vi "GetVIByName.vi"(0 "Application Ref in":refnum<vi>, 5 "VI Name":string, 7 "Timeout(5 sec)":dbl=5.0, 11 "error in (no error)":errorcluster) -> (4 "Application Ref out":refnum<vi>, 6 "VI Reference":refnum<vi>, 15 "error out":errorcluster)   [LabVIEW 2016, in "Drona.lvlib" / "GetVI.lvlib"]
doc: "Gives the reference of the specified VI given by VI name as input."
uses:
  GetVI.lvlib
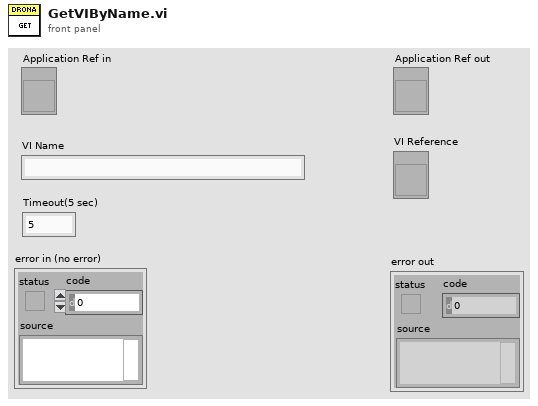
[diagram p1: front panel]
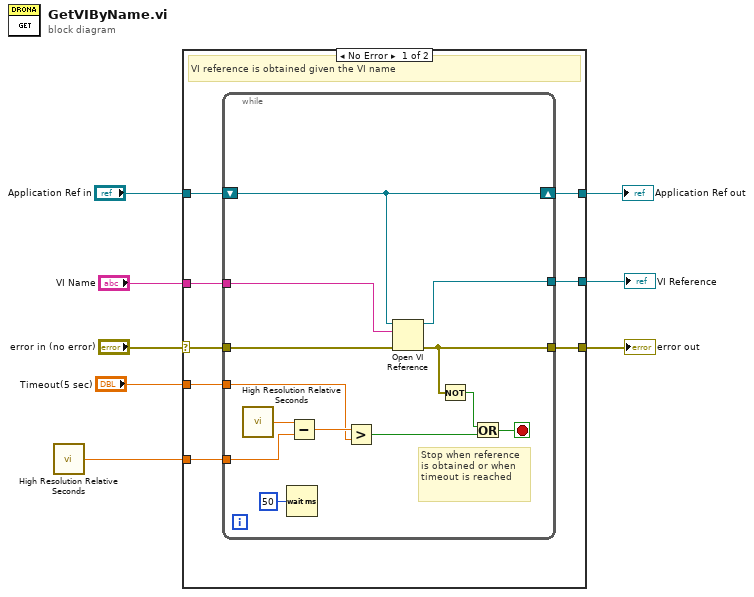
[diagram p0: block diagram]
diagram:
  n1 = call <vilib>:"High Resolution Relative Seconds.vi"() -> ("relative seconds"=w1:dbl)
  n2 = case shown="No Error" "error in (no error)" {
    selector: "error in (no error)" -> [w16 w31]
    tunnel: [w15 w31] -> w7
    tunnel: [w9 w30] -> w5
    tunnel: "Application Ref in" -> [w10 w30]
    tunnel: "VI Name" -> [w13 _]
    tunnel: [w14 _] -> w3
    tunnel: "Timeout(5 sec)" -> [w12 _]
    tunnel: w1 -> [w11 _]
    frame No Error {
      # "VI reference is obtained given the VI name"
      n3 = while {
        tunnel: [w22] -> w14
        tunnel: w13 -> [w28]
        tunnel: w12 -> [w24]
        tunnel: w11 -> [w26]
        tunnel: w16 -> [w29]
        tunnel: [w21] -> w15
        shift-right: [w17] -> w9
        shift-left: w10 -> [w17]
        stop <- w18 stop-if-true
        # "Stop when reference is obtained or when timeout is reached"
        n4 = call <vilib>:"High Resolution Relative Seconds.vi"() -> ("relative seconds"=w27:dbl)
        n5 = Wait (ms)(milliseconds to wait=u32 50) -> ()  [unwired: 1 out]
        n6 = Subtract(x=w27, y=w26) -> (x-y=w25:dbl)
        n7 = Greater?(x=w25, y=w24) -> (0:w19:bool)
        n8 = Open VI Reference(application reference (local)=w17, vi path=w28, error in (no error)=w29) -> (vi reference=w22:refnum<vi>, error out=w21:errorcluster)  [unwired: 3 in]
        n9 = Not(x=w21) -> (.not. x?=w20:bool)
        n10 = Or(x=w20, y=w19) -> (x .or. y?=w18:bool)
      }
    }
    frame Error {
    }
  }
  "error out" <- w7
  "Application Ref out" <- w5
  "VI Reference" <- w3
